vi "KeithleyReset.vi"(8 "error in":errorcluster, 10 "address (16)":i16=16, 11 "bus (0)":i32) -> (0 "error out":errorcluster)   [LabVIEW 2017]
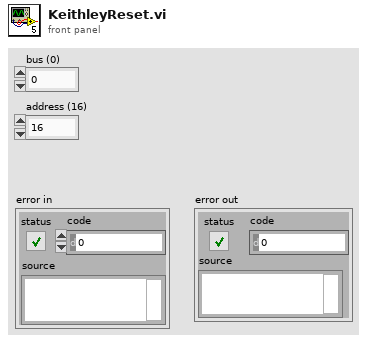
[diagram p1: front panel]
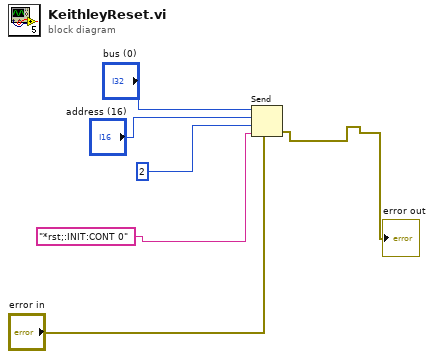
[diagram p0: block diagram]
diagram:
  n1 = Send(0:"bus (0)", 2:"address (16)", 3:i16 2 ("mode"), 4:"error in", 5:"*rst;:INIT:CONT 0" ("data string")) -> (8:→"error out":errorcluster)  [unwired: 2 out]
